vi "Build_Actuation_Array.vi"(0 "Actuation Seq 1":string, 1 "Seq1_Enable":bool, 2 "Seq2_Enable":bool, 5 "Actuation Seq 2":string, 7 "Actuation Seq 3":string, 9 "Actuation Seq 4":string, 11 "error in (no error)":errorcluster, 12 "Seq3_Enable":bool, 13 "Seq4_Enable":bool) -> (6 "Array Out":i32[](array[numeric]), 15 "error out":errorcluster)   [LabVIEW 2017]
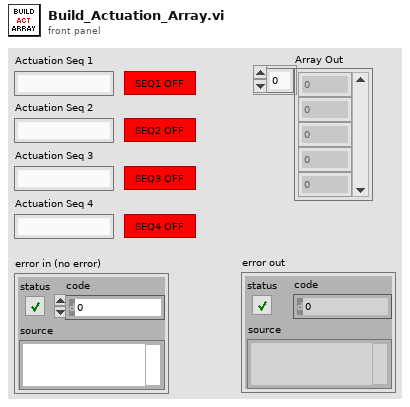
[diagram p1: front panel]
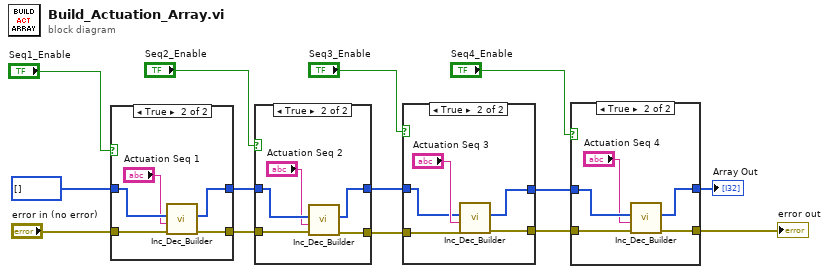
[diagram p0: block diagram]
diagram:
  n1 = case shown="True" "Seq1_Enable" {
    tunnel: "error in (no error)" -> [w16 w21]
    tunnel: [w16 w20] -> w10
    tunnel: i32[] [] ("Array In") -> [w15 w19]
    tunnel: [w15 w17] -> w9
    frame False {
    }
    frame True {
      n2 = call "Inc_Dec_Builder.vi"("error in (no error)"=w21, "Index_Str_In"="Actuation Seq 1", "Array In"=w19) -> ("error out"=w20:errorcluster, "Array"=w17:i32[])  [unwired: 7 in]
    }
  }
  n3 = case shown="True" "Seq2_Enable" {
    tunnel: w10 -> [w22 w28]
    tunnel: [w22 w27] -> w8
    tunnel: w9 -> [w23 w26]
    tunnel: [w23 w24] -> w6
    frame False {
    }
    frame True {
      n4 = call "Inc_Dec_Builder.vi"("error in (no error)"=w28, "Index_Str_In"="Actuation Seq 2", "Array In"=w26) -> ("error out"=w27:errorcluster, "Array"=w24:i32[])  [unwired: 7 in]
    }
  }
  n5 = case shown="True" "Seq3_Enable" {
    tunnel: w8 -> [w29 w35]
    tunnel: [w29 w34] -> w4
    tunnel: w6 -> [w30 w32]
    tunnel: [w30 w31] -> w3
    frame False {
    }
    frame True {
      n6 = call "Inc_Dec_Builder.vi"("error in (no error)"=w35, "Index_Str_In"="Actuation Seq 3", "Array In"=w32) -> ("error out"=w34:errorcluster, "Array"=w31:i32[])  [unwired: 7 in]
    }
  }
  n7 = case shown="True" "Seq4_Enable" {
    tunnel: w4 -> [w36 w41]
    tunnel: w3 -> [w37 w42]
    tunnel: [w36 w40] -> w2
    tunnel: [w37 w39] -> w1
    frame False {
    }
    frame True {
      n8 = call "Inc_Dec_Builder.vi"("error in (no error)"=w41, "Index_Str_In"="Actuation Seq 4", "Array In"=w42) -> ("error out"=w40:errorcluster, "Array"=w39:i32[])  [unwired: 7 in]
    }
  }
  "error out" <- w2
  "Array Out" <- w1
